vi "gentec-M-Link.Set Trigger Polarity.vi"(0 "VISA resource In":refnum<visa-resource-name>, 2 "Trigger Polarity":T1 items=["Falling Edge", "Rising Edge"], 5 "error in (no error)":errorcluster) -> (11 "Data Read":string, 13 "Read Timeout":bool, 14 "VISA resource Out":refnum<visa-resource-name>, 16 "Success":bool, 19 "error out":errorcluster)   [LabVIEW 2014, in "gentec-M-Link - Driver.lvlib"]
doc: "Data to write: pol0 or pol1\n\nSets the external trigger polarity for energy or radiometric measurement. pol0 is rising edge, pol1 is falling edge (the other way round than what is described in M-Link User's Manual, Revision 1.0)."
uses:
  gentec-M-Link - Driver.lvlib
  Type Defs/gentec-M-Link.Trigger Polarity.ctl
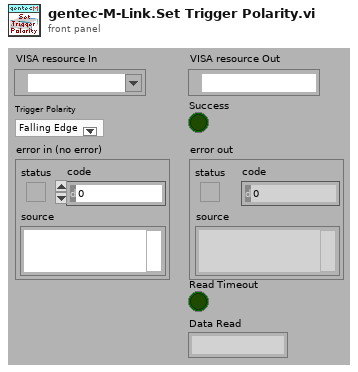
[diagram p1: front panel]
types:
  T1 = typedef "gentec-M-Link - Driver.lvlib/gentec-M-Link.Trigger Polarity.ctl" = u16
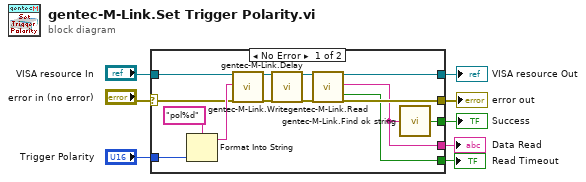
[diagram p0: block diagram]
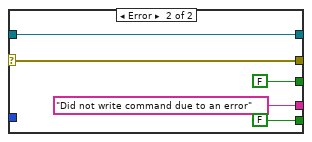
[diagram p2: hidden frame]
diagram:
  n1 = case shown="No Error" "error in (no error)" {
    selector: "error in (no error)" -> [w15 w27]
    tunnel: [w16 w27] -> w7
    tunnel: "VISA resource In" -> [w14 w26]
    tunnel: [w13 w26] -> w5
    tunnel: "Trigger Polarity" -> [w12 _]
    tunnel: [w11 FALSE ("Found")] -> w3
    tunnel: [w10 "Did not write command due to an error" ("Data Read")] -> w2
    tunnel: [w9 FALSE ("Read Timeout")] -> w1
    frame No Error {
      n2 = Format Into String(format string="pol%d", w12) -> (resulting string=w21:string)  [unwired: 2 in, 1 out]
      n3 = call "gentec-M-Link.Write.vi"("VISA resource (In)"=w14, "Data To Write"=w21, "error in (no error)"=w15) -> ("VISA resource (Out)"=w17:refnum<visa-resource-name>, "error out"=w18:errorcluster)  [unwired: 14 in, 1 out]
      n4 = call "gentec-M-Link.Delay.vi"("VISA resource In"=w17, "error in (no error)"=w18) -> ("VISA resource Out"=w20:refnum<visa-resource-name>, "error out"=w19:errorcluster)  [unwired: 16 in]
      n5 = call "gentec-M-Link.Read.vi"("VISA resource (In)"=w20, "error in (no error)"=w19) -> ("VISA resource (Out)"=w13:refnum<visa-resource-name>, "Data Read"=w10:string, "Read Timeout"=w9:bool, "error out"=w16:errorcluster)  [unwired: 13 in, 1 out]
      n6 = call "gentec-M-Link.Find ok string.vi"("string"=w10) -> ("Found"=w11:bool)
    }
    frame Error {
    }
  }
  "error out" <- w7
  "VISA resource Out" <- w5
  "Success" <- w3
  "Data Read" <- w2
  "Read Timeout" <- w1
